vi "e.gate RealTimeClock.vi"(0 "Configuration  in":T2, 3 "e.gate Time in":T1, 7 "error in (no error)":errorcluster, 11 "Enable writing":bool) -> (20 "Configuration out":T2, 23 "e.gate Time out":T1, 27 "error out":errorcluster)   [LabVIEW 2016]
uses:
  e.gate Configuration.ctl
  e.gate Channel Data.ctl
  e.gate Data Type.ctl
  e.gate Protocol Type.ctl
  e.gate Module  Data.ctl
  e.gateHSP_DLLhandle.ctl
  e.gate Time.ctl
panel:
  out "verknüpfter String":string
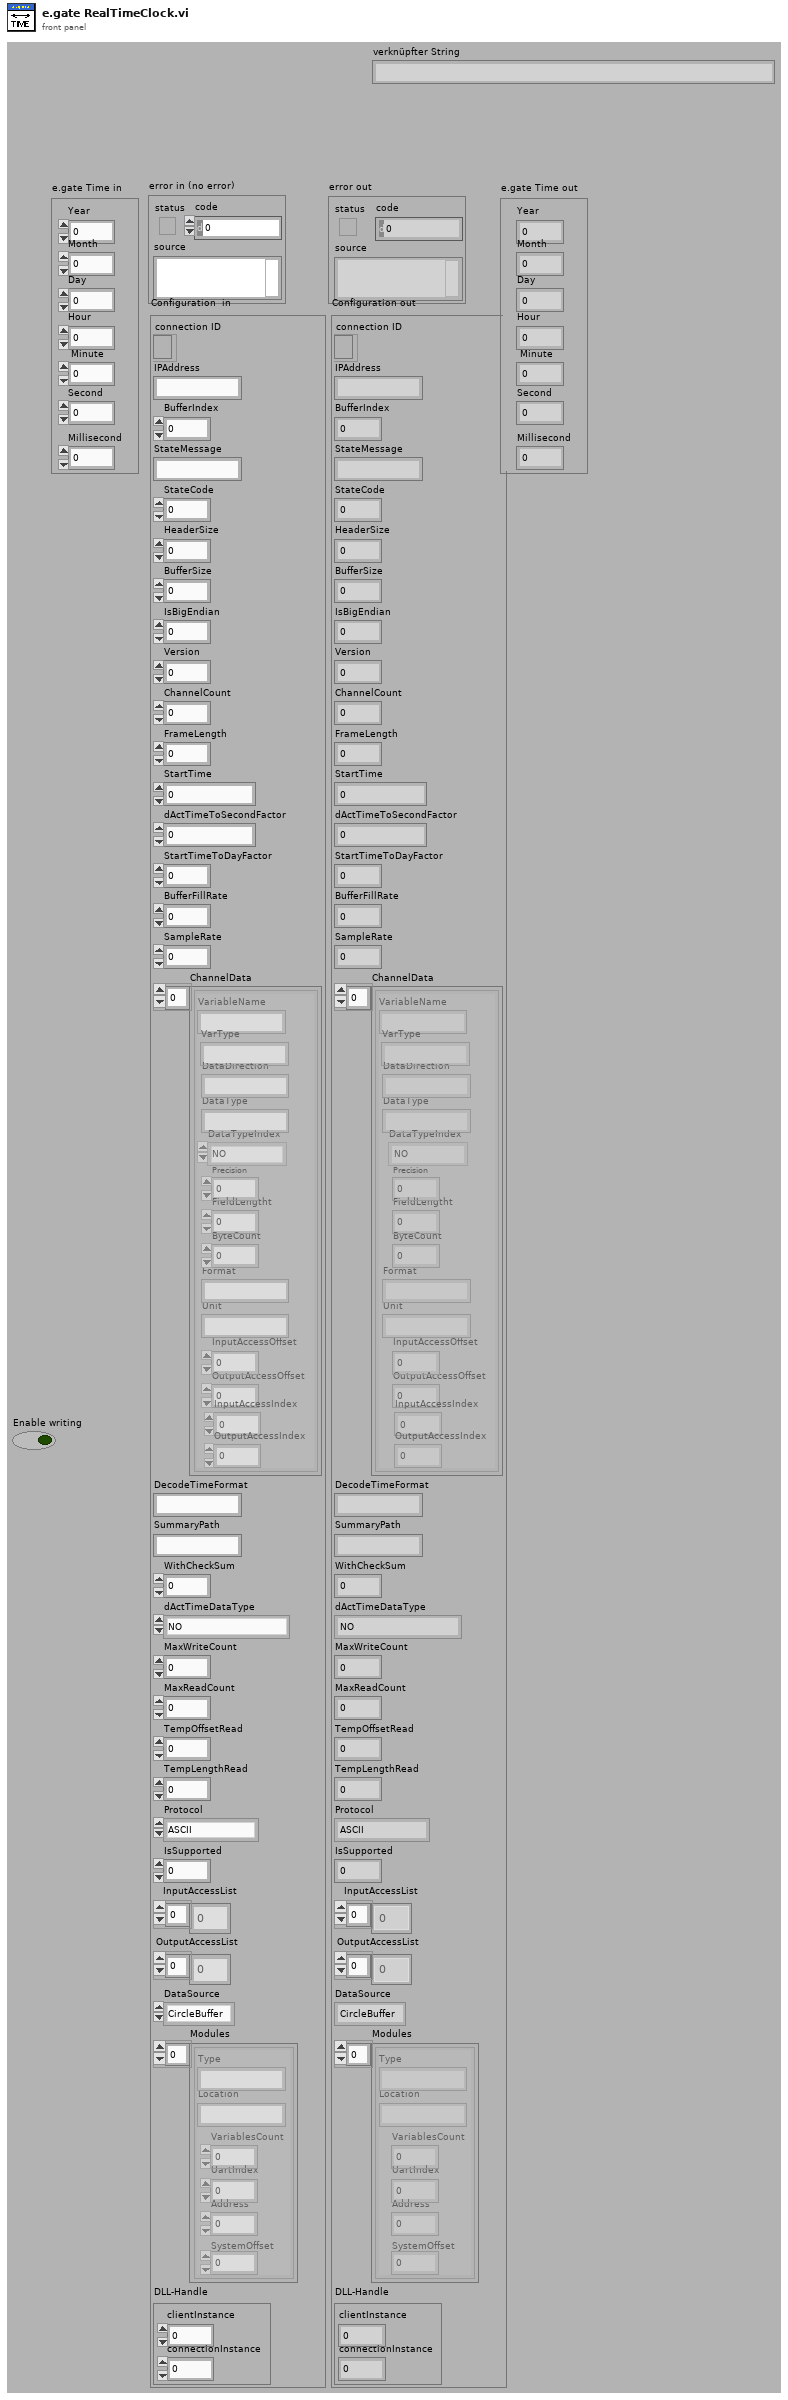
[diagram p1: front panel]
types:
  T1 = typedef "e.gate Time.ctl" = cluster{"Year":dbl, "Month":dbl, "Day":dbl, "Hour":dbl, " Minute":dbl, "Second":dbl, "Millisecond":dbl}
  T2 = typedef "e.gate Configuration.ctl" = cluster{"connection ID":refnum<k5>, "IPAddress":string, "BufferIndex":i32, "StateMessage":string, "StateCode":i8, "HeaderSize":i32, "BufferSize":i32, "IsBigEndian":i32, "Version":i32, "ChannelCount":i32, "FrameLength":i32, "StartTime":dbl, "dActTimeToSecondFactor":dbl, "StartTimeToDayFactor":dbl, "BufferFillRate":dbl, "SampleRate":dbl, "ChannelData":T3[], "DecodeTimeFormat":string, "SummaryPath":string, "WithCheckSum":i32, "dActTimeDataType":T4, "MaxWriteCount":i32, "MaxReadCount":i32, "TempOffsetRead":i32, "TempLengthRead":i32, "Protocol":T5, "IsSupported":i32, "InputAccessList":i32[], "OutputAccessList":i32[], "DataSource":enum16{"CircleBuffer", "test.con Logger", "test.con Archive"}, "Modules":T6[], "DLL-Handle":T7}
  T3 = typedef "e.gate Channel Data.ctl" = cluster{"VariableName":string, "DataDirection":string, "DataType":string, "DataTypeIndex":T4, "Precision":i16, "FieldLengtht":i16, "ByteCount":i32, "Format":string, "Unit":string, "InputAccessOffset":i32, "OutputAccessOffset":i16, "InputAccessIndex":i16, "OutputAccessIndex":i16, "VarType":string}
  T4 = typedef "e.gate Data Type.ctl" = enum16{"NO", "BOOL", "SINT8", "USINT8", "SINT16", "USINT16", "SINT32", "USINT32", "FLOAT", "SET8", "SET16", "SET32", "DOUBLE", "SINT64", "USINT64", "SET64"}
  T5 = typedef "e.gate Protocol Type.ctl" = enum16{"ASCII", "HighspeedPort Online", "HighspeedPort Buffer", "eGateHighspeedPortDLL "}
  T6 = typedef "e.gate Module  Data.ctl" = cluster{"Type":string, "Location":string, "VariablesCount":i16, "UartIndex":i16, "Address":i16, "SystemOffset":i16}
  T7 = typedef "e.gateHSP_DLLhandle.ctl" = cluster{"clientInstance":i32, "connectionInstance":i32}
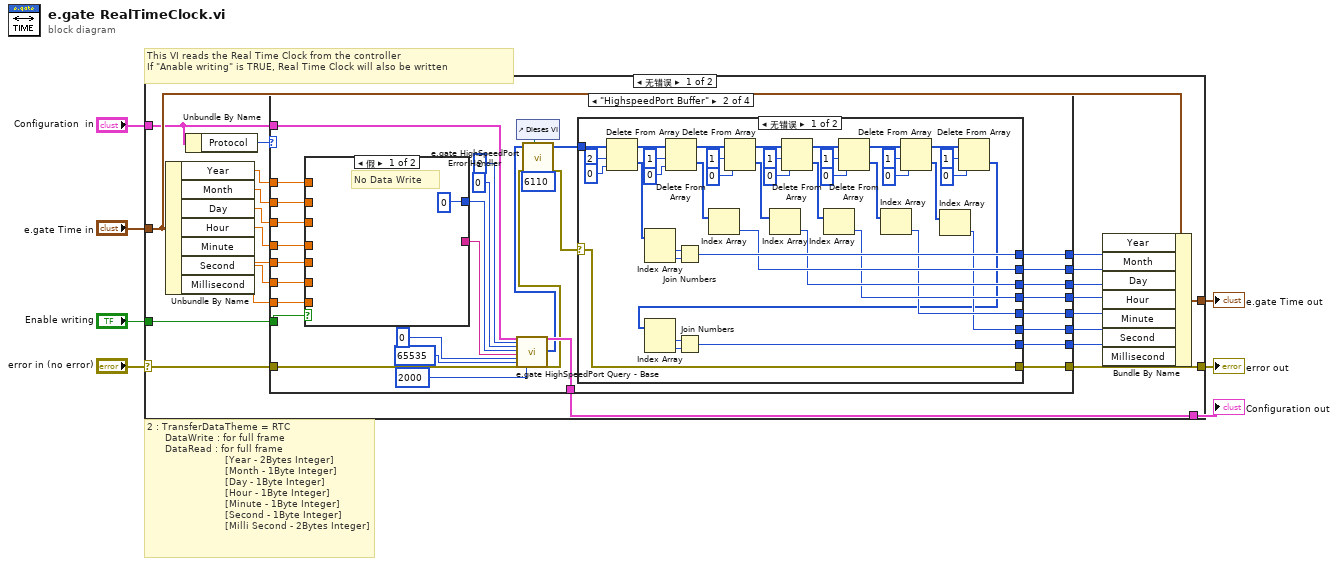
[diagram p0: block diagram]
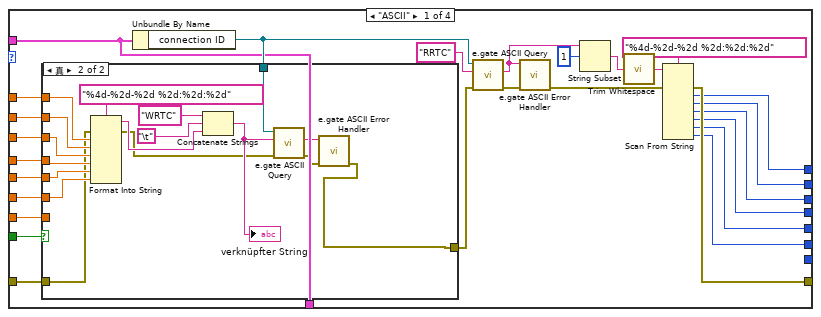
[diagram p2: hidden frame]
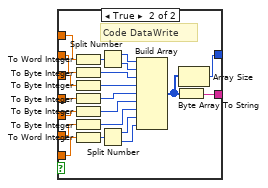
[diagram p5: hidden frame]
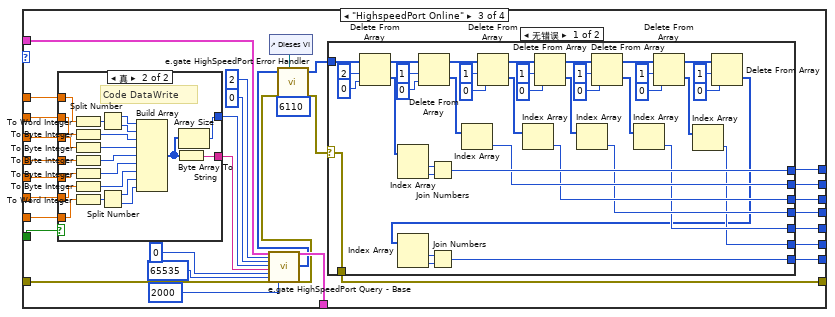
[diagram p6: hidden frame]
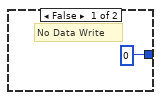
[diagram p8: hidden frame]
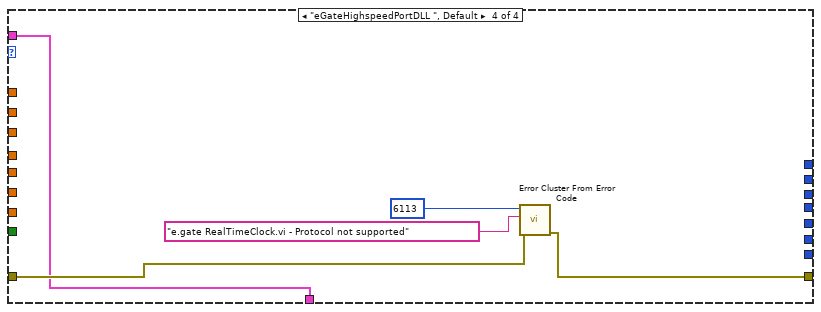
[diagram p9: hidden frame]
diagram:
  # "This VI reads the Real Time Clock from the controller \nIf \"Anable writing\" is TRUE, Real Time Clock will also be written"
  # "2 : TransferDataTheme = RTC\n      DataWrite : for full frame\n      DataRead : for full frame\n\t                         [Year - 2Bytes Integer]\n                          [Month - 1Byte Integer]\n                          [Day - 1Byte Integer]\n                          [Hour - 1Byte Integer]\n                          [Minute - 1Byte Integer]\n                          [Second - 1Byte Integer]\n                          [Milli Second - 2Bytes Integer]"
  n1 = case shown="无错误" "error in (no error)" {
    selector: "error in (no error)" -> [w28 w270]
    tunnel: [w29 w270] -> w7
    tunnel: "Configuration  in" -> [w8 w271]
    tunnel: [w9 w271] -> w4
    tunnel: "Enable writing" -> [w27 _]
    tunnel: [w18 _] -> w2
    tunnel: "e.gate Time in" -> [w10 _]
    frame No Error {
      n2 = Unbundle By Name(w10) -> ("Year"=w25:dbl, "Month"=w24:dbl, "Day"=w23:dbl, "Hour"=w22:dbl, "Minute"=w21:dbl, "Second"=w20:dbl, "Millisecond"=w19:dbl)
      n3 = Unbundle By Name(w8) -> ("Protocol"=w26:T5)
      n4 = case shown="\"HighspeedPort Buffer\"" w26 {
        tunnel: [w49 w77 w174 w266] -> w29
        tunnel: w28 -> [w47 w106 w201 w267]
        tunnel: w27 -> [w46 w100 w197 _]
        tunnel: w25 -> [w45 w99 w196 _]
        tunnel: w24 -> [w44 w98 w195 _]
        tunnel: w23 -> [w43 w97 w194 _]
        tunnel: w22 -> [w42 w96 w193 _]
        tunnel: w21 -> [w41 w95 w192 _]
        tunnel: w20 -> [w40 w94 w191 _]
        tunnel: w19 -> [w39 w93 w190 _]
        tunnel: w8 -> [w31 w83 w179 w265]
        tunnel: [w32 w90 w181 _] -> w17
        tunnel: [w33 w89 w182 _] -> w16
        tunnel: [w34 w88 w183 _] -> w15
        tunnel: [w35 w87 w184 _] -> w14
        tunnel: [w37 w86 w185 _] -> w13
        tunnel: [w36 w85 w186 _] -> w12
        tunnel: [_ w84 w187 _] -> w11
        tunnel: [w31 w82 w180 w265] -> w9
        frame "ASCII" {
          n5 = Unbundle By Name(w31) -> ("connection ID"=w38:refnum<k5>)
          n6 = case shown="真" w46 {
            tunnel: w47 -> [w57 w67]
            tunnel: w45 -> [_ w74]
            tunnel: w44 -> [_ w73]
            tunnel: w43 -> [_ w72]
            tunnel: w42 -> [_ w71]
            tunnel: w41 -> [_ w70]
            tunnel: w40 -> [_ w69]
            tunnel: w39 -> [_ _]
            tunnel: w38 -> [_ w59]
            tunnel: [w57 w58] -> w30
            frame False {
            }
            frame True {
              n7 = Format Into String(format string="%4d-%2d-%2d %2d:%2d:%2d", error in=w67, w74, w73, w72, w71, w70, w69) -> (resulting string=w61:string, error out=w60:errorcluster)  [unwired: 1 in]
              n8 = Concatenate Strings("WRTC" ("format string"), "\t" ("Tabulatorkonstante"), w61) -> (w66:string)
              "verknüpfter String" <- w66
              n9 = call "e.gate ASCII Query.vi"("error in (no error)"=w60, "Command"=w66, "connection ID In"=w59) -> ("error out"=w62:errorcluster, "Response"=w63:string)  [unwired: 7 out]
              n10 = call "e.gate ASCII Error Handler.vi"("error in (no error)"=w62, "String"=w63) -> ("error out"=w58:errorcluster)  [unwired: 9 out]
            }
          }
          n11 = call "e.gate ASCII Query.vi"("error in (no error)"=w30, "Command"="RRTC" ("format string"), "connection ID In"=w38) -> ("error out"=w55:errorcluster, "Response"=w56:string)  [unwired: 7 out]
          n12 = call "e.gate ASCII Error Handler.vi"("error in (no error)"=w55, "String"=w56) -> ("error out"=w48:errorcluster)  [unwired: 9 out]
          n13 = String Subset(string=w56, offset (0)=1) -> (substring=w53:string)  [unwired: 1 out]
          n14 = call <vilib>:"Trim Whitespace.vi"("string"=w53) -> ("trimmed string"=w50:string)  [unwired: 1 in]
          n15 = Scan From String(format string="%4d-%2d-%2d %2d:%2d:%2d", input string=w50, error in=w48) -> (error out=w49:errorcluster, output 1=w32:i32, output 2=w33:i32, output 3=w34:i32, output 4=w35:i32, output 5=w37:i32, output 6=w36:i32)  [unwired: 1 in, 8 out]
        }
        frame "HighspeedPort Buffer" {
          n16 = case shown="假" w100 {
            tunnel: [0 ("LengthWrite") w150] -> w101
            tunnel: w99 -> [_ w157]
            tunnel: w98 -> [_ w156]
            tunnel: w97 -> [_ w155]
            tunnel: w96 -> [_ w154]
            tunnel: w95 -> [_ w153]
            tunnel: w94 -> [_ w152]
            tunnel: w93 -> [_ w151]
            tunnel: [_ w149] -> w92
            frame False {
              # "No Data Write"
            }
            frame True {
              # "Code DataWrite"
              n17 = To Word Integer(number=w157) -> (16bit integer=w158:i16)
              n18 = To Byte Integer(number=w156) -> (8bit integer=w161:i8)
              n19 = To Byte Integer(number=w155) -> (8bit integer=w162:i8)
              n20 = To Byte Integer(number=w154) -> (8bit integer=w163:i8)
              n21 = To Byte Integer(number=w153) -> (8bit integer=w164:i8)
              n22 = To Byte Integer(number=w152) -> (8bit integer=w165:i8)
              n23 = To Word Integer(number=w151) -> (16bit integer=w166:i16)
              n24 = Split Number(x=w158) -> (hi(x)=w159:u8, lo(x)=w160:u8)
              n25 = Split Number(x=w166) -> (hi(x)=w167:u8, lo(x)=w168:u8)
              n26 = Build Array(w159, w160, w161, w162, w163, w164, w165, w167, w168) -> (w169:u8[])
              n27 = Byte Array To String(unsigned byte array=w169) -> (string=w149:string)
              n28 = Array Size(array=w169) -> (size(s)=w150:i32)
            }
          }
          n29 = control-ref of="Dieses VI"() -> (w75:refnum<vi>)
          n30 = call "e.gate HighSpeedPort Query - Base.vi"("e.gate Configuration in"=w83, "Command"=2, "OffsetWrite"=0, "LengthWrite"=w101, "DataWrite"=w92, "OffsetRead"=0, "LengthRead"=65535, "error in (no error)"=w106, "Timeout (1000)"=2000) -> ("e.gate Configuration out"=w82:T2, "Data (out binary)"=w81:u8[], "error out"=w79:errorcluster)  [unwired: 1 in, 15 out]
          n31 = call "e.gate HighSpeedPort Error Handler.vi"("error code start index"=6110, "VI reference"=w75, "error in (no error)"=w79, "binary data in"=w81) -> ("error out"=w78:errorcluster, "binary out"=w80:u8[])  [unwired: 6 out]
          n32 = case shown="无错误" w78 {
            selector: w78 -> [w107 w147]
            tunnel: [w146 _] -> w90
            tunnel: [w145 _] -> w89
            tunnel: [w144 _] -> w88
            tunnel: [w143 _] -> w87
            tunnel: [w142 _] -> w86
            tunnel: [w141 _] -> w85
            tunnel: [w140 _] -> w84
            tunnel: w80 -> [w139 _]
            tunnel: [w107 w147] -> w77
            frame No Error {
              n33 = Delete From Array(array=w139, length=2 ("Länge"), index=0 ("Index")) -> (deleted portion=w135:u8[], array with subset deleted=w136:u8[])
              n34 = Index Array(array=w135) -> (element #1=w134:u8, element #2=w133:u8)  [unwired: 2 in]
              n35 = Delete From Array(array=w136, length=1 ("Länge"), index=0 ("Index")) -> (deleted portion=w124:u8[], array with subset deleted=w130:u8[])
              n36 = Join Numbers(hi=w134, lo=w133) -> ((hi.lo)=w146:u16)
              n37 = Index Array(array=w124) -> (element=w145:u8)  [unwired: 1 in]
              n38 = Delete From Array(array=w130, length=1 ("Länge"), index=0 ("Index")) -> (deleted portion=w123:u8[], array with subset deleted=w125:u8[])
              n39 = Index Array(array=w123) -> (element=w144:u8)  [unwired: 1 in]
              n40 = Delete From Array(array=w125, length=1 ("Länge"), index=0 ("Index")) -> (deleted portion=w122:u8[], array with subset deleted=w119:u8[])
              n41 = Index Array(array=w122) -> (element=w143:u8)  [unwired: 1 in]
              n42 = Delete From Array(array=w119, length=1 ("Länge"), index=0 ("Index")) -> (deleted portion=w118:u8[], array with subset deleted=w115:u8[])
              n43 = Index Array(array=w118) -> (element=w142:u8)  [unwired: 1 in]
              n44 = Delete From Array(array=w115, length=1 ("Länge"), index=0 ("Index")) -> (deleted portion=w114:u8[], array with subset deleted=w111:u8[])
              n45 = Index Array(array=w114) -> (element=w141:u8)  [unwired: 1 in]
              n46 = Delete From Array(array=w111, length=1 ("Länge"), index=0 ("Index")) -> (deleted portion=w108:u8[])  [unwired: 1 out]
              n47 = Index Array(array=w108) -> (element #1=w110:u8, element #2=w109:u8)  [unwired: 2 in]
              n48 = Join Numbers(hi=w110, lo=w109) -> ((hi.lo)=w140:u16)
            }
            frame Error {
            }
          }
        }
        frame "HighspeedPort Online" {
          n49 = case shown="真" w197 {
            tunnel: [0 ("LengthWrite") w245] -> w198
            tunnel: w196 -> [_ w252]
            tunnel: w195 -> [_ w251]
            tunnel: w194 -> [_ w250]
            tunnel: w193 -> [_ w249]
            tunnel: w192 -> [_ w248]
            tunnel: w191 -> [_ w247]
            tunnel: w190 -> [_ w246]
            tunnel: [_ w244] -> w189
            frame False {
              # "No Data Write"
            }
            frame True {
              # "Code DataWrite"
              n50 = To Word Integer(number=w252) -> (16bit integer=w253:i16)
              n51 = To Byte Integer(number=w251) -> (8bit integer=w256:i8)
              n52 = To Byte Integer(number=w250) -> (8bit integer=w257:i8)
              n53 = To Byte Integer(number=w249) -> (8bit integer=w258:i8)
              n54 = To Byte Integer(number=w248) -> (8bit integer=w259:i8)
              n55 = To Byte Integer(number=w247) -> (8bit integer=w260:i8)
              n56 = To Word Integer(number=w246) -> (16bit integer=w261:i16)
              n57 = Split Number(x=w253) -> (hi(x)=w254:u8, lo(x)=w255:u8)
              n58 = Split Number(x=w261) -> (hi(x)=w262:u8, lo(x)=w263:u8)
              n59 = Build Array(w254, w255, w256, w257, w258, w259, w260, w262, w263) -> (w264:u8[])
              n60 = Byte Array To String(unsigned byte array=w264) -> (string=w244:string)
              n61 = Array Size(array=w264) -> (size(s)=w245:i32)
            }
          }
          n62 = call "e.gate HighSpeedPort Query - Base.vi"("e.gate Configuration in"=w179, "Command"=2, "OffsetWrite"=0, "LengthWrite"=w198, "DataWrite"=w189, "OffsetRead"=0, "LengthRead"=65535, "error in (no error)"=w201, "Timeout (1000)"=2000) -> ("e.gate Configuration out"=w180:T2, "Data (out binary)"=w177:u8[], "error out"=w175:errorcluster)  [unwired: 1 in, 15 out]
          n63 = control-ref of="Dieses VI"() -> (w173:refnum<vi>)
          n64 = call "e.gate HighSpeedPort Error Handler.vi"("error code start index"=6110, "VI reference"=w173, "error in (no error)"=w175, "binary data in"=w177) -> ("error out"=w176:errorcluster, "binary out"=w172:u8[])  [unwired: 6 out]
          n65 = case shown="无错误" w176 {
            selector: w176 -> [w202 w242]
            tunnel: [w227 _] -> w181
            tunnel: [w225 _] -> w182
            tunnel: [w223 _] -> w183
            tunnel: [w221 _] -> w184
            tunnel: [w216 _] -> w185
            tunnel: [w215 _] -> w186
            tunnel: [w205 _] -> w187
            tunnel: w172 -> [w203 _]
            tunnel: [w202 w242] -> w174
            frame No Error {
              n66 = Delete From Array(array=w203, length=2 ("Länge"), index=0 ("Index")) -> (deleted portion=w238:u8[], array with subset deleted=w239:u8[])
              n67 = Index Array(array=w238) -> (element #1=w237:u8, element #2=w236:u8)  [unwired: 2 in]
              n68 = Delete From Array(array=w239, length=1 ("Länge"), index=0 ("Index")) -> (deleted portion=w226:u8[], array with subset deleted=w233:u8[])
              n69 = Join Numbers(hi=w237, lo=w236) -> ((hi.lo)=w227:u16)
              n70 = Index Array(array=w226) -> (element=w225:u8)  [unwired: 1 in]
              n71 = Delete From Array(array=w233, length=1 ("Länge"), index=0 ("Index")) -> (deleted portion=w224:u8[], array with subset deleted=w228:u8[])
              n72 = Index Array(array=w224) -> (element=w223:u8)  [unwired: 1 in]
              n73 = Delete From Array(array=w228, length=1 ("Länge"), index=0 ("Index")) -> (deleted portion=w222:u8[], array with subset deleted=w218:u8[])
              n74 = Index Array(array=w222) -> (element=w221:u8)  [unwired: 1 in]
              n75 = Delete From Array(array=w218, length=1 ("Länge"), index=0 ("Index")) -> (deleted portion=w217:u8[], array with subset deleted=w212:u8[])
              n76 = Index Array(array=w217) -> (element=w216:u8)  [unwired: 1 in]
              n77 = Delete From Array(array=w212, length=1 ("Länge"), index=0 ("Index")) -> (deleted portion=w211:u8[], array with subset deleted=w208:u8[])
              n78 = Index Array(array=w211) -> (element=w215:u8)  [unwired: 1 in]
              n79 = Delete From Array(array=w208, length=1 ("Länge"), index=0 ("Index")) -> (deleted portion=w204:u8[])  [unwired: 1 out]
              n80 = Index Array(array=w204) -> (element #1=w207:u8, element #2=w206:u8)  [unwired: 2 in]
              n81 = Join Numbers(hi=w207, lo=w206) -> ((hi.lo)=w205:u16)
            }
            frame Error {
            }
          }
        }
        frame "eGateHighspeedPortDLL ", Default {
          n82 = call <vilib>:"Error Cluster From Error Code.vi"("error in (no error)"=w267, "error message (\"\")"="e.gate RealTimeClock.vi - Protocol not supported" ("error message (\"\")"), "error code (0)"=i16 6113 ("y")) -> ("error out"=w266:errorcluster)  [unwired: 1 in, 5 out]
        }
      }
      n83 = Bundle By Name(cluster=w10, "Year"=w17, "Month"=w16, "Day"=w15, "Hour"=w14, "Minute"=w13, "Second"=w12, "Millisecond"=w11) -> (w18:T1)
    }
    frame Error {
    }
  }
  "error out" <- w7
  "Configuration out" <- w4
  "e.gate Time out" <- w2
